vi "Init Local Reconfig VI.vi"(8 "error in (no error)":errorcluster, 9 "Config Channels":dbl[](array[numeric]), 10 "IOV ref":refnum<k21>, 11 "Module DVR":refnum<data-value>) -> (0 "error out":errorcluster, 3 "Local Reconfig VI Ref":refnum<vi>)   [LabVIEW 2020, in "SEECD Engine.lvlib"]
uses:
  SEECD Engine.lvlib
  <vilib>/NI VeriStand/Custom Device Tools/Custom Device Utility Library/Custom Device Utility Library.lvlib
  Includes/Modules.lvlibp/RSI Module/RSI Module.lvclass
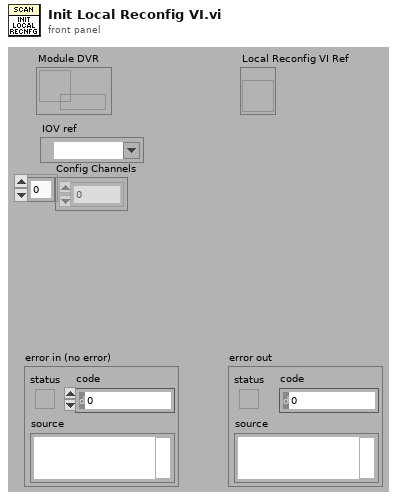
[diagram p1: front panel]
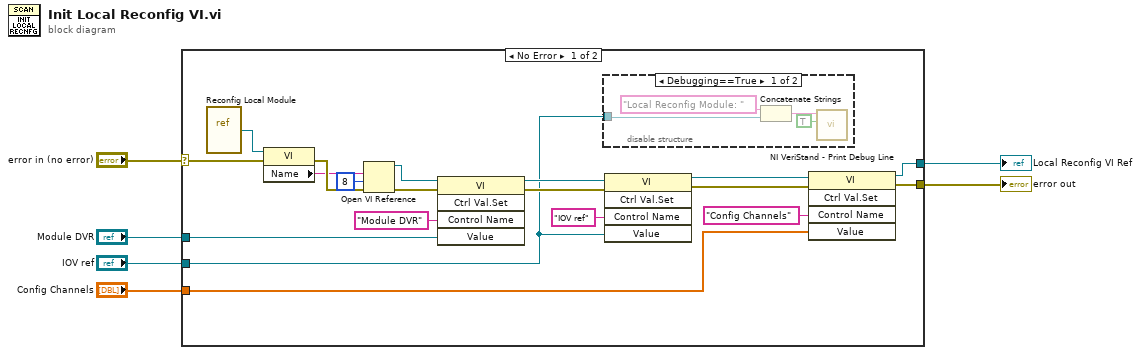
[diagram p0: block diagram]
diagram:
  n1 = case shown="No Error" "error in (no error)" {
    selector: "error in (no error)" -> [w8 w30]
    tunnel: "Module DVR" -> [w25 _]
    tunnel: "IOV ref" -> [w7 _]
    tunnel: "Config Channels" -> [w11 _]
    tunnel: [w10 _] -> w3
    tunnel: [w9 w30] -> w2
    frame No Error {
      n2 = vi-ref "Reconfig Local Module.vi"() -> (w22:refnum<vi>)
      n3 = property class="VI"(reference=w22, error in=w8) -> (error out=w23:errorcluster, "Name"=w20:string)  [unwired: 1 out]
      n4 = Open VI Reference(vi path=w20, options=8, error in (no error)=w23) -> (vi reference=w24:refnum<vi>, error out=w21:errorcluster)  [unwired: 3 out]
      n5 = invoke class="VI" method="Ctrl Val.Set"(reference=w24, error in=w21, "Control Name"="Module DVR", "Value"=w25) -> (reference out=w16:refnum<vi>, error out=w15:errorcluster)  [unwired: 1 in, 3 out]
      n6 = disable-structure shown="Debugging==True" {
        disable-tunnel: w7 -> [w28 _]
        frame condition #0 {
          n7 = Concatenate Strings("Local Reconfig Module: ", w28) -> (w27:string)
          n8 = call <vilib>:"NI VeriStand - Print Debug Line.vi"("Add to log file? (F)"=TRUE, "Message"=w27) -> ()  [unwired: 9 in, 1 out]
        }
        frame condition #1 (active) {
        }
      }
      n9 = invoke class="VI" method="Ctrl Val.Set"(reference=w16, error in=w15, "Control Name"="IOV ref", "Value"=w7) -> (reference out=w12:refnum<vi>, error out=w13:errorcluster)  [unwired: 1 in, 3 out]
      n10 = invoke class="VI" method="Ctrl Val.Set"(reference=w12, error in=w13, "Control Name"="Config Channels", "Value"=w11) -> (reference out=w10:refnum<vi>, error out=w9:errorcluster)  [unwired: 1 in, 3 out]
    }
    frame Error {
    }
  }
  "Local Reconfig VI Ref" <- w3
  "error out" <- w2
